vi "srednia.vi"() -> ()   [LabVIEW 2022 SP3]
uses:
  <vilib>/numeric/Random Number (Range) I64.vi
  <vilib>/numeric/sub_Random U32.vi
panel:
  out "Srednia":dbl
  out "Liczby":dbl[](array[numeric])
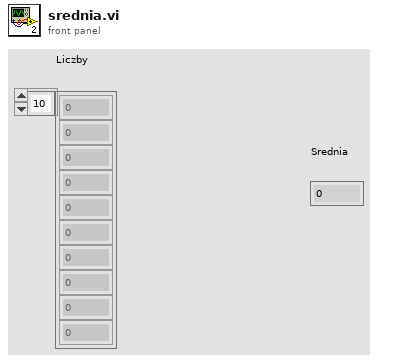
[diagram p1: front panel]
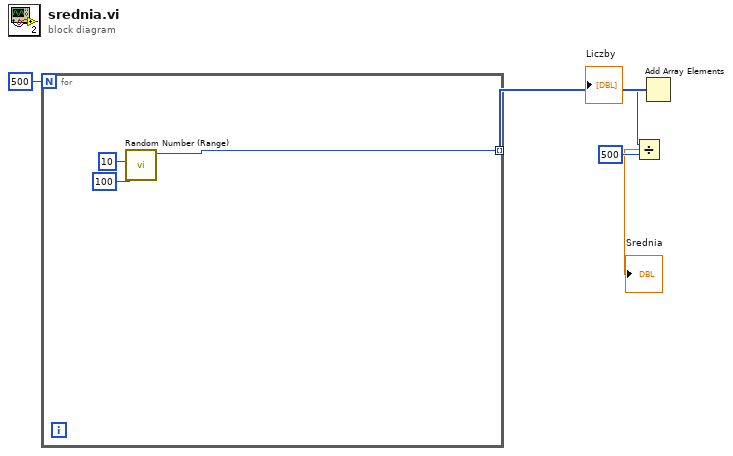
[diagram p0: block diagram]
diagram:
  n1 = for {
    N: 500 -> [_]
    tunnel: [w6] -> w4 mode=indexing
    n2 = call-poly <vilib>:"Random Number (Range).vi"("lower bound (-100)"=u64 10 ("lower bound (0)"), "upper bound (100)"=u64 100) -> ("number"=w6:i64)  [unwired: 9 in]
  }
  "Liczby" <- w4
  n3 = Add Array Elements(numeric array=w4) -> (sum=w3:i64)
  n4 = Divide(x=w3, y=i64 500) -> (x/y=→"Srednia":dbl)
